vi "Initialize.vi"(8 "error in (no error)":errorcluster, 9 "Reset (True)":bool=TRUE, 10 "ID Query (True)":bool=TRUE, 11 "VISA resource name":refnum<visa-resource-name>) -> (0 "error out":errorcluster, 3 "VISA resource name out":refnum<visa-resource-name>)   [LabVIEW 2023, in "Stanford Research 830.lvlib"]
doc: "Establishes communication with the instrument and optionally performs an instrument identification query and/or an instrument reset. It also places the instrument in a default state needed for other instrument driver operations. Therefore, call this VI before calling other instrument driver VIs for this instrument. Generally, you need to call the Initialize VI only once at the beginning of an application."
uses:
  Stanford Research 830.lvlib
panel:
  # "(c) 2006 National Instruments.  ALL RIGHTS RESERVED."
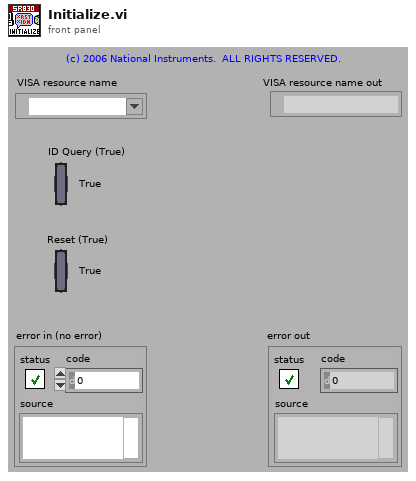
[diagram p1: front panel]
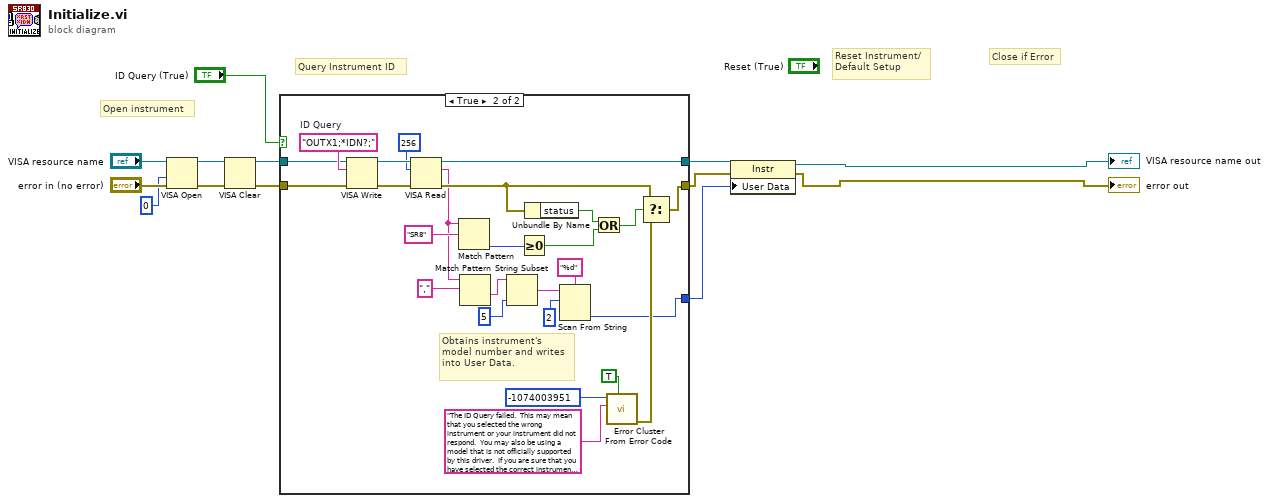
[diagram p0: block diagram]
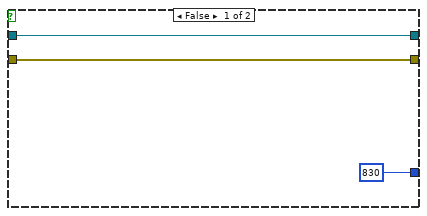
[diagram p2: hidden frame]
diagram:
  # "Close if Error"
  # "Query Instrument ID"
  # "Reset Instrument/\nDefault Setup"
  # "Open instrument"
  n1 = VISA Open(access mode=u32 0, error in (no error)="error in (no error)", VISA resource name="VISA resource name") -> (VISA resource name=w9:refnum<visa-resource-name>, error out=w8:errorcluster)  [unwired: 2 in]
  n2 = VISA Clear(VISA resource name=w9, error in (no error)=w8) -> (VISA resource name out=w7:refnum<visa-resource-name>, error out=w6:errorcluster)
  n3 = case shown="True" "ID Query (True)" {
    tunnel: [w15 w42] -> w3
    tunnel: [w16 w41] -> w4
    tunnel: w7 -> [w16 w26]
    tunnel: w6 -> [w15 w25]
    tunnel: [830 w17] -> w5
    frame False {
    }
    frame True {
      w36 = "OUTX1;*IDN?;"  # ID Query
      # "Obtains instrument's model number and writes into User Data."
      n4 = VISA Write(VISA resource name=w26, write buffer=w36, error in (no error)=w25) -> (VISA resource name out=w40:refnum<visa-resource-name>, error out=w39:errorcluster)  [unwired: 1 out]
      n5 = VISA Read(VISA resource name=w40, byte count=u32 256, error in (no error)=w39) -> (VISA resource name out=w41:refnum<visa-resource-name>, read buffer=w21:string, error out=w30:errorcluster)  [unwired: 1 out]
      n6 = Match Pattern(string=w21, regular expression="SR8") -> (offset past match=w31:i32)  [unwired: 1 in, 3 out]
      n7 = Match Pattern(string=w21, regular expression=",") -> (after substring=w22:string)  [unwired: 1 in, 3 out]
      n8 = String Subset(string=w22, length (rest)=5 ("length (rest)")) -> (substring=w20:string)  [unwired: 1 in]
      n9 = Greater Or Equal To 0?(x=w31) -> (x >= 0?=w28:bool)
      n10 = Unbundle By Name(w30) -> ("status"=w29:bool)
      n11 = Scan From String(format string="%d", input string=w20, initial scan location=2 ("offset")) -> (output 1=w17:i32)  [unwired: 2 in, 3 out]
      n12 = Or(x=w29, y=w28) -> (x .or. y?=w27:bool)
      n13 = call <vilib>:"Error Cluster From Error Code.vi"("show call chain? (False)"=TRUE, "error message (\"\")"="The ID Query failed.  This may mean that you selected the wrong instrument or your instrument did not respond.  You may also be using a model that is not officially supported by this driver.  If you are sure that you have selected the correct instrument and it is responding, try disabling the ID Query." ("Source (VI Name)"), "error code (0)"=-1074003951 ("Code")) -> ("error out"=w35:errorcluster)  [unwired: 6 in]
      n14 = Select(t=w30, s=w27, f=w35) -> (s? t:f=w42:errorcluster)
    }
  }
  n15 = property class="Instr"(reference=w4, error in=w3, "User Data"=w5) -> (reference out=→"VISA resource name out":refnum<visa-resource-name>, error out=→"error out":errorcluster)
